vi "Query Available SN List.vi"(8 "error in (no error)":errorcluster, 11 "MC switch refnum in":refnum<k24>) -> (0 "error out":errorcluster, 2 "serial number list":string[](array[string]), 3 "MC switch refnum out":refnum<k24>)   [LabVIEW 2019, in "Minicircuit RF Switch Box.lvlib"]
doc: "Returns the internal temperature (in degrees Celsius) measured at 1 of the internal sensors (model dependent):\n\n- USB-1SPDT-A18 / RC-1SPDT-A18 (1 sensor)\n- USB-1SP4T-A18 / RC-1SP4T-A18 (1 sensor)\n- RC-2MTS-18 (2 sensors)\n- USB-2SPDT-A18 / RC-2SPDT-A18 (2 sensors)\n- USB-3SPDT-A18 / RC-3SPDT-A18 (2 sensors)\n- USB-4SPDT-A18 / RC-4SPDT-A18 (2 sensors)\n- USB-8SPDT-A18 / RC-8SPDT-A18 (3 sensors)\n- RC-2SP4T-x (2 sensors)\n- RC-2SP6T-A12 (2 sensors)\n\nNote: Units with serial numbers earlier than 11108010000 may have a different number of\nsensors than indicated above.\n\nIf a sensor that does not exist is polled (for example there is no sensor 2 on USB-1SPDT-A18)\nthe temperature returned will be “+25.00”"
uses:
  <instrlib>/LV_Minicircuit_RF_Switch/Minicircuit RF Switch Box.lvlib
  C:/Program Files (x86)/National Instruments/LabVIEW 2019/instr.lib/LV_Minicircuit_RF_Switch/mcl_RF_Switch_Controller_NET45.dll
  mcl_RF_Switch_Controller_NET45.dll
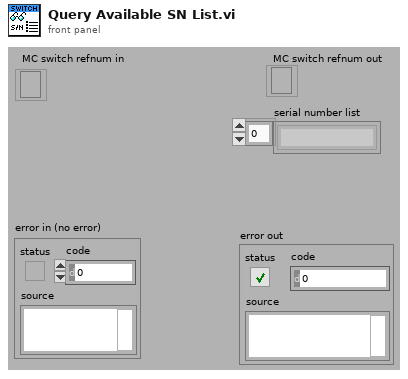
[diagram p1: front panel]
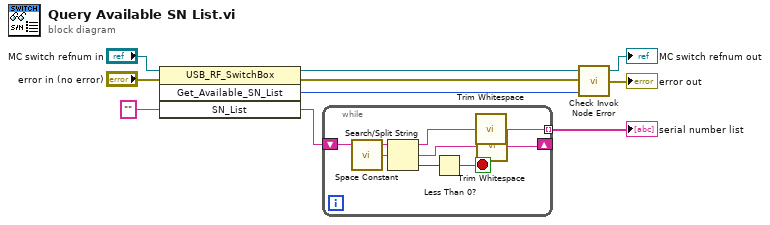
[diagram p0: block diagram]
diagram:
  n1 = invoke class="USB_RF_SwitchBox" method="Get_Available_SN_List"(reference="MC switch refnum in", error in="error in (no error)", "SN_List"="" ("Add_List")) -> (reference out=w8:refnum<k24>, error out=w7:errorcluster, "Get_Available_SN_List"=w6:i32, "SN_List"=w3:string)  [unwired: 1 in]
  n2 = while {
    shift-right: [w12] -> _
    shift-left: w3 -> [w18]
    tunnel: [w17] -> w2 mode=indexing
    stop <- w13 stop-if-true
    n3 = call <vilib>:"Space Constant.vi"() -> ("String"=w15:string)
    n4 = Search/Split String(string=w18, search string/char (-)=w15) -> (substring before match=w16:string, match + rest of string=w11:string, offset of match=w14:i32)  [unwired: 1 in]
    n5 = Less Than 0?(x=w14) -> (x < 0?=w13:bool)
    n6 = call <vilib>:"Trim Whitespace.vi"("string"=w16) -> ("trimmed string"=w17:string)  [unwired: 1 in]
    n7 = call <vilib>:"Trim Whitespace.vi"("string"=w11) -> ("trimmed string"=w12:string)  [unwired: 1 in]
  }
  "serial number list" <- w2
  n8 = call <instrlib>:"Check Invok Node Error.vi"("Connect"=w6, "error in (no error)"=w7, "MC switch refnum in"=w8) -> ("error out"=→"error out":errorcluster, "MC switch refnum out"=→"MC switch refnum out":refnum<k24>)  [unwired: 1 in]
